vi "send serial command.vi"() -> ()   [LabVIEW 2017]
uses:
  typedefs/commandType.ctl
panel:
  in  "Command":T1
  out "error out":errorcluster
  out "VISA resource name out":refnum<visa-resource-name>
  in  "data":dbl[](array[numeric])
  in  "time (s)":dbl
  in  "error in (no error)":errorcluster
  in  "visa resource":refnum<visa-resource-name>
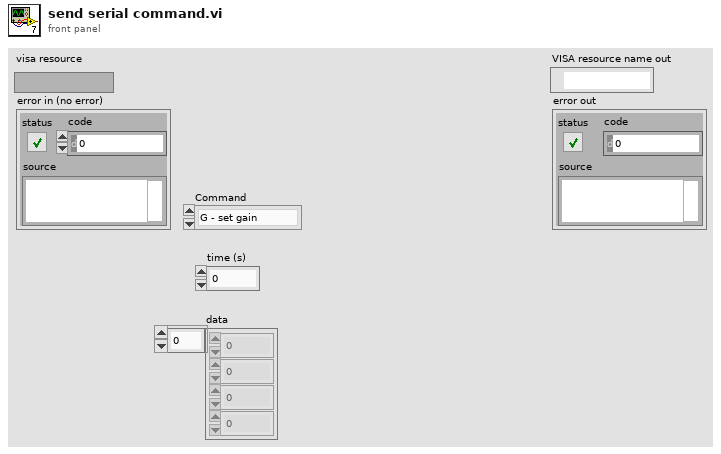
[diagram p1: front panel]
types:
  T1 = typedef "commandType.ctl" = enum16{"G - set gain", "C - activate coil", "D - deactivate coil", "L - set LED", "A - set AUTO", "V - set verbose"}
  T2 = cluster{"data[0]":dbl, "data[1]":dbl, "data[2]":dbl, "data[3]":dbl}
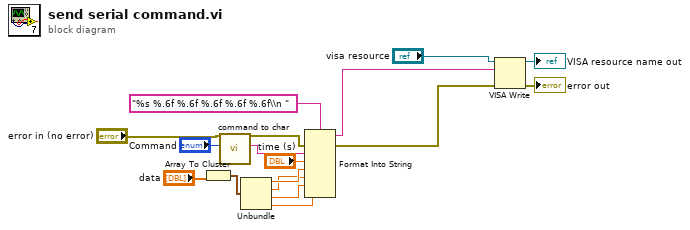
[diagram p0: block diagram]
diagram:
  n1 = Array To Cluster(array="data") -> (cluster=w11:T2)
  n2 = call "command to char.vi"("Command"="Command") -> ("char"=w14:string)  [unwired: 10 in]
  n3 = Unbundle(w11) -> ("data[0]"=w10:dbl, "data[1]"=w9:dbl, "data[2]"=w8:dbl, "data[3]"=w7:dbl)
  n4 = Format Into String(format string="%s %.6f %.6f %.6f %.6f %.6f\\n ", error in="error in (no error)", w14, "time (s)", w10, w9, w8, w7) -> (resulting string=w6:string, error out=w4:errorcluster)  [unwired: 1 in]
  n5 = VISA Write(VISA resource name="visa resource", write buffer=w6, error in (no error)=w4) -> (VISA resource name out=→"VISA resource name out":refnum<visa-resource-name>, error out=→"error out":errorcluster)  [unwired: 1 out]
